vi "Initialize Camera and CheckList.vi"(11 "ListBox in":refnum<vi>) -> (0 "Cluster 2":T1, 1 "Cluster":T2, 2 "Array":cluster{string[]}[](array[cluster]), 3 "File Refnum":T3)   [LabVIEW 2016]
uses:
  <vilib>/Utility/config.llb/Config Data RefNum.ctl
  <vilib>/Utility/config.llb/Read Key (String).vi
  <vilib>/Utility/config.llb/Read Key (I32).vi
  <vilib>/Utility/config.llb/NI_LVConfig.lvlib
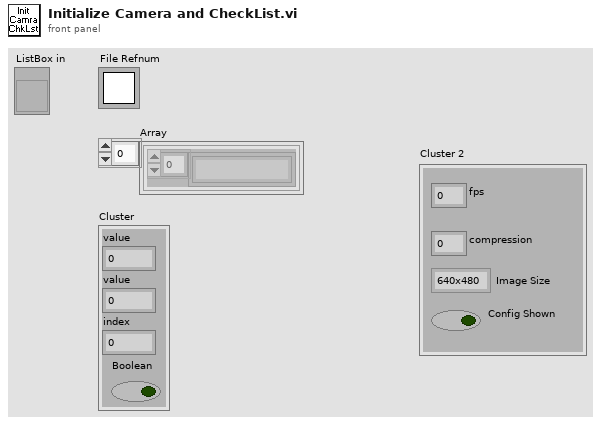
[diagram p1: front panel]
types:
  T1 = cluster{"compression":i32, "fps":i32, "Image Size":enum16{"640x480", "320x240", "160x120"}, "Config Shown":bool}
  T2 = cluster{"value":i32, "value":i32, "index":i32, "Boolean":bool}
  T3 = typedef "NI_LVConfig.lvlib/Config Data RefNum.ctl" = refnum<k1>
  T4 = cluster{"value":i32, "value":i32, "index":i32, bool}
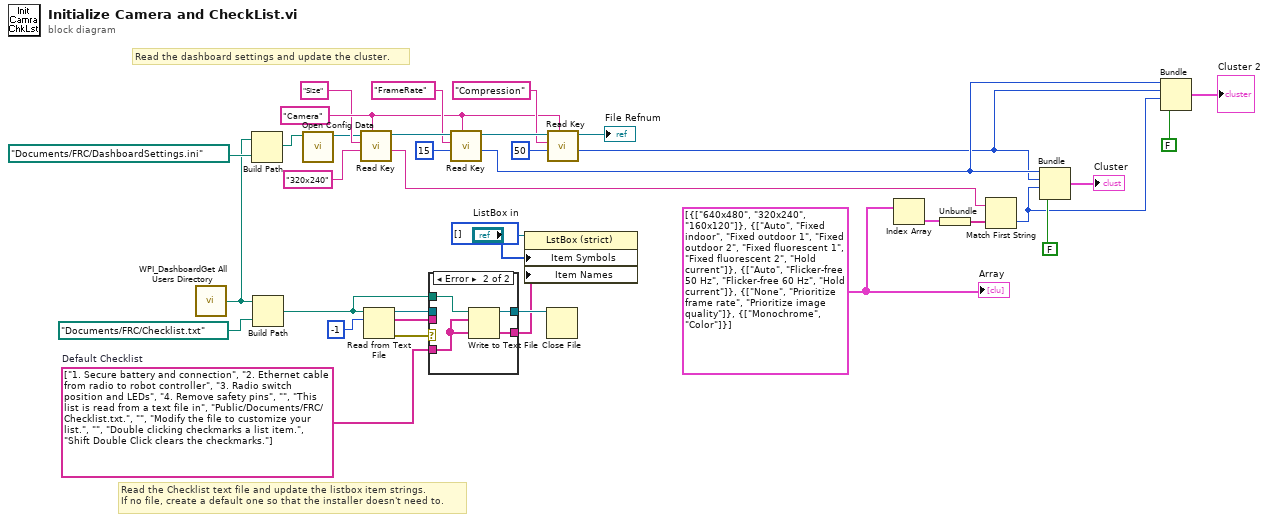
[diagram p0: block diagram]
diagram:
  w21 = "Camera"
  w27 = cluster{string[]}[] [{["640x480", "320x240", "160x120"]}, {["Auto", "Fixed indoor", "Fixed outdoor 1", "Fixed outdoor 2", "Fixed fluorescent 1", "Fixed fluorescent 2", "Hold current"]}, {["Auto", "Flicker-free 50 Hz", "Flicker-free 60 Hz", "Hold current"]}, {["None", "Prioritize frame rate", "Prioritize image quality"]}, {["Monochrome", "Color"]}]
  w14 = string[] ["1. Secure battery and connection", "2. Ethernet cable from radio to robot controller", "3. Radio switch position and LEDs", "4. Remove safety pins", "", "This list is read from a text file in", "Public/Documents/FRC/Checklist.txt.", "", "Modify the file to customize your list.", "", "Double clicking checkmarks a list item.", "Shift Double Click clears the checkmarks."]  # Default Checklist
  # "Read the Checklist text file and update the listbox item strings.\nIf no file, create a default one so that the installer doesn't need to."
  # "Read the dashboard settings and update the cluster."
  n1 = call <vilib>:"WPI_DashboardGet All Users Directory.vi"() -> ("All User Path"=w16:path)
  n2 = Build Path(base path=w16, name or relative path=path "Documents/FRC/DashboardSettings.ini") -> (appended path=w17:path)
  n3 = Build Path(base path=w16, name or relative path=path "Documents/FRC/Checklist.txt") -> (appended path=w13:path)
  n4 = call <vilib>:"Open Config Data.vi"("configuration file path"=w17) -> ("refnum"=w18:T3)  [unwired: 8 in, 2 out]
  n5 = call-poly <vilib>:"Read Key.vi"("section"=w21, "default value"="320x240", "key"="Size", "refnum"=w18) -> ("value"=w29:string, "refnum out"=w33:T3)  [unwired: 2 in, 4 out]
  n6 = Read from Text File(file (use dialog)=w13, count=-1 ("timeout ms (25000)")) -> (refnum out=w31:refnum<file>, text=w12:string[], error out=w11:errorcluster)  [unwired: 2 in, 1 out]
  n7 = case shown="Error" w11 {
    tunnel: w12 -> [w38 _]
    tunnel: [w38 w40] -> w15
    tunnel: w14 -> [_ w40]
    tunnel: w13 -> [_ w41]
    tunnel: [w37 w39] -> w32
    tunnel: w31 -> [w37 _]
    frame No Error {
    }
    frame Error {
      n8 = Write to Text File(file (use dialog)=w41, text=w40) -> (refnum out=w39:refnum<file>)  [unwired: 2 in, 2 out]
    }
  }
  n9 = call-poly <vilib>:"Read Key.vi"("section"=w21, "default value"=15, "key"="FrameRate", "refnum"=w33) -> ("value"=w2:i32, "refnum out"=w34:T3)  [unwired: 1 in, 5 out]
  n10 = property on="Property Node" class="LstBox (strict)"(reference="ListBox in", "Item Symbols"=i32[] [], "Item Names"=w15) -> ()  [unwired: 1 in, 2 out]
  n11 = Close File(refnum=w32) -> ()  [unwired: 1 in, 2 out]
  n12 = call-poly <vilib>:"Read Key.vi"("section"=w21, "default value"=50, "key"="Compression", "refnum"=w34) -> ("value"=w1:i32, "refnum out"=→"File Refnum":T3)  [unwired: 1 in, 5 out]
  n13 = Index Array(array=w27) -> (element=w26:cluster{string[]})  [unwired: 1 in]
  n14 = Unbundle(w26) -> (w28:string[])
  n15 = Match First String(2:w28, 3:w29) -> (0:w4:i32)  [unwired: 1 out]
  n16 = Bundle("value"=w2, "value"=w1, "index"=w4, FALSE) -> (→"Cluster":T4)  [unwired: 1 out]
  n17 = Bundle("value"=w2, "value"=w1, "index"=w4, FALSE) -> (→"Cluster 2":T4)  [unwired: 1 in]
  "Array" <- w27
